vi "Get Executable Attributes.vi"(8 "error in (no error)":errorcluster, 11 "Executable in":refnum<class "Executable.lvclass">) -> (0 "error out":errorcluster, 2 "Executable Attributes":T1, 3 "Executable out":refnum<class "Executable.lvclass">)   [LabVIEW 2023, in "HAF.lvlib" / "Executable.lvclass"]
doc: "Provides a set of attributes that are used to control how the Driver should run the Executable on an Instrument."
uses:
  Executable.lvclass
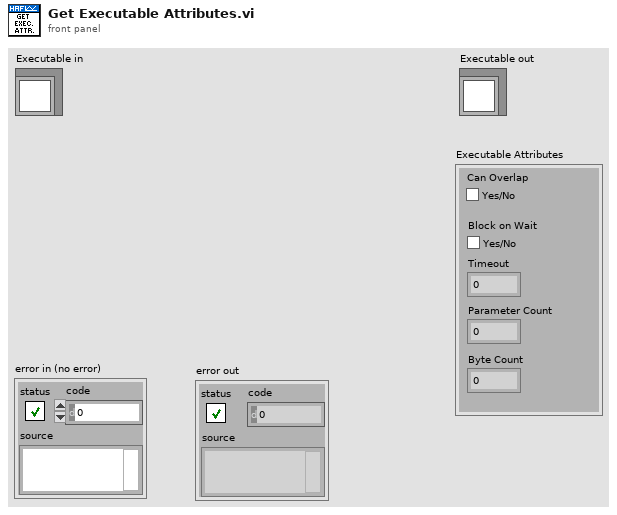
[diagram p1: front panel]
types:
  T1 = cluster{"Can Overlap":bool, "Block on Wait":bool, "Timeout":u32, "Byte Count":u32, "Parameter Count":u32}
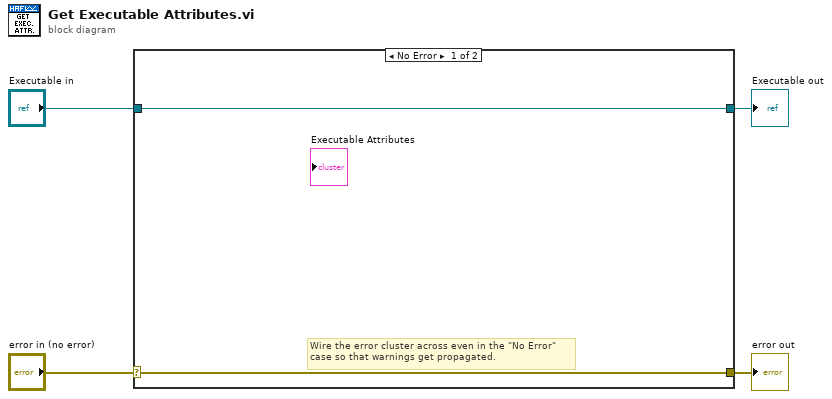
[diagram p0: block diagram]
diagram:
  n1 = case shown="No Error" "error in (no error)" {
    selector: "error in (no error)" -> [w5 w8]
    tunnel: [w5 w8] -> w3
    tunnel: [w6 w7] -> w1
    tunnel: "Executable in" -> [w6 w7]
    frame No Error {
      # "Wire the error cluster across even in the \"No Error\"\ncase so that warnings get propagated."
    }
    frame Error {
    }
  }
  "error out" <- w3
  "Executable out" <- w1
